vi "Window-Simple Timelapse Player.vi"() -> ()   [LabVIEW 2013]
uses:
  User Interface/Visualisation/Timelapse Viewer/Typedefs/Custom slider-vertical.ctl
  User Interface/Visualisation/Timelapse Viewer/Typedefs/Timelapse viewer refs.ctl
  <vilib>/Utility/miscctls.llb/LVPointTypeDef.ctl
  User Interface/Visualisation/Timelapse Viewer/Typedefs/Speed Viewer States enum.ctl
  Typedefs/Save-Load enum.ctl
  User Interface/Visualisation/Functional Imaging Viewer/Typedefs/Get-Set-Clear Control.ctl
  User Interface/Visualisation/Timelapse Viewer/Typedefs/Select Play-Stop button to show.ctl
  <vilib>/vision/Image Controls.llb/IMAQ Image.ctl
  User Interface/Visualisation/Timelapse Viewer/Globals/gl_Time series viewer globals.vi
  Global Variables/General Globals.vi
panel:
  in  "Intensity":T1={-4095.0, 4095.0} scale=0.0..4095.0
  in  "Back":bool
  in  "Play":bool
  in  "Stop":bool
  in  "Colour":u16(ring)=2 items=["Gray", "Red", "Green"]
  out "Image":T2(plugin-control)
  in  "AVI File Path":path
  out "Speed Graph":dbl[](graph) caption="Speed Chart"
  out "Export data subset":bool
  out "Export vid":bool
  out "Stop (ind)":bool
  in  "Scrollbar":i32(c297)
  out "Speed Profile Graph":dbl[](graph)
  # "<-- Available through the menu"
  # "<-- Available through the menu"
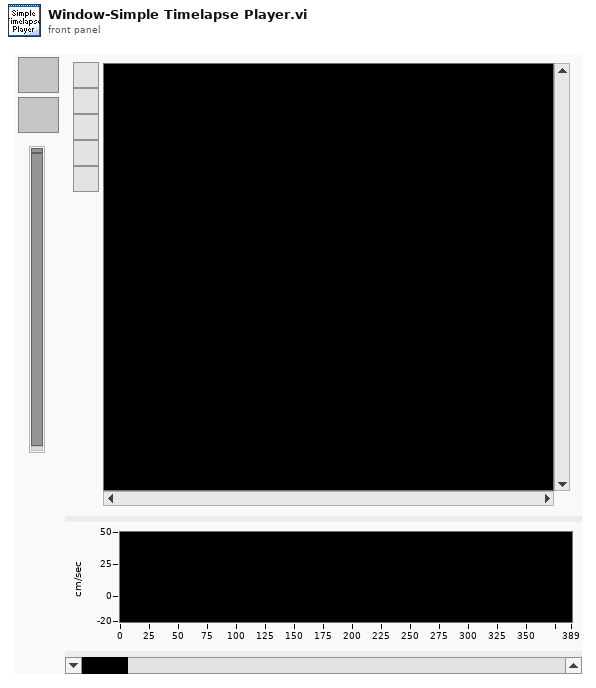
[diagram p1: front panel]
types:
  T1 = typedef "Custom slider-vertical.ctl" = cluster{dbl, dbl}
  T2 = typedef "IMAQ Image.ctl" = refnum<image>
  T3 = typedef "Timelapse viewer refs.ctl" = cluster{"This VI":refnum<vi>, "AVI Mode ind":refnum<vi>, "Play":refnum<vi>, "Stop":refnum<vi>, "Back":refnum<vi>, "Scrollbar":refnum<vi>, "Video length info":refnum<vi>, "Expected speed values":refnum<vi>, "Intensity":refnum<vi>, "Path":refnum<vi>, "Selection sliders":refnum<vi>, "Speed Graph ref":refnum<vi>, "Frame rate set (fps)":refnum<vi>}
  T4 = typedef "LVPointTypeDef.ctl" = cluster{"Horizontal":i16, "Vertical":i16}
  T5 = typedef "Save-Load enum.ctl" = enum16{"Save to file", "Load from file", "Compare from file"}
  T6 = typedef "Speed Viewer States enum.ctl" = enum16{"Idle", "Initialise", "Playback", "Scroll bar event", "Speed cursor event", "Back to start", "Exit"}
  T7 = typedef "Image Type" = u32
  T8 = typedef "Custom slider-horisontal.ctl" = cluster{dbl, dbl}
  T9 = typedef "Select Play-Stop button to show.ctl" = enum16{"Show Play button", "Show Stop button"}
  T10 = cluster{"Conversion Method":u32, "Minimum Value":i32, "Maximum Value":i32, "Number Of Shifts":i32}
  T11 = typedef "AVI modes refs cluster.ctl" = cluster{"AVI1 ref":T12, "AVI2 refs":T13[], "AVI # frames":u32[]}
  T12 = typedef "AviRefnum.ctl" = refnum<k1>
  T13 = typedef "IMAQ AVI2 Refnum.ctl" = refnum<k20>
  T14 = typedef "AVI implementation enum.ctl" = enum16{"AVI1", "AVI2"}
  T15 = cluster{"# of frames to export":i32, "Initial frame's owning file":T13, "8-bit AVI file path":path, "Cursors location":cluster{"Number of first frame":i32, "Number of last frame":i32}}
  T16 = typedef "Get-Set-Clear Control.ctl" = enum16{"Get", "Set", "Clear"}
  T17 = typedef "Speed graph behaviour enum.ctl" = enum16{"Scrolling data", "Scrolling cursor"}
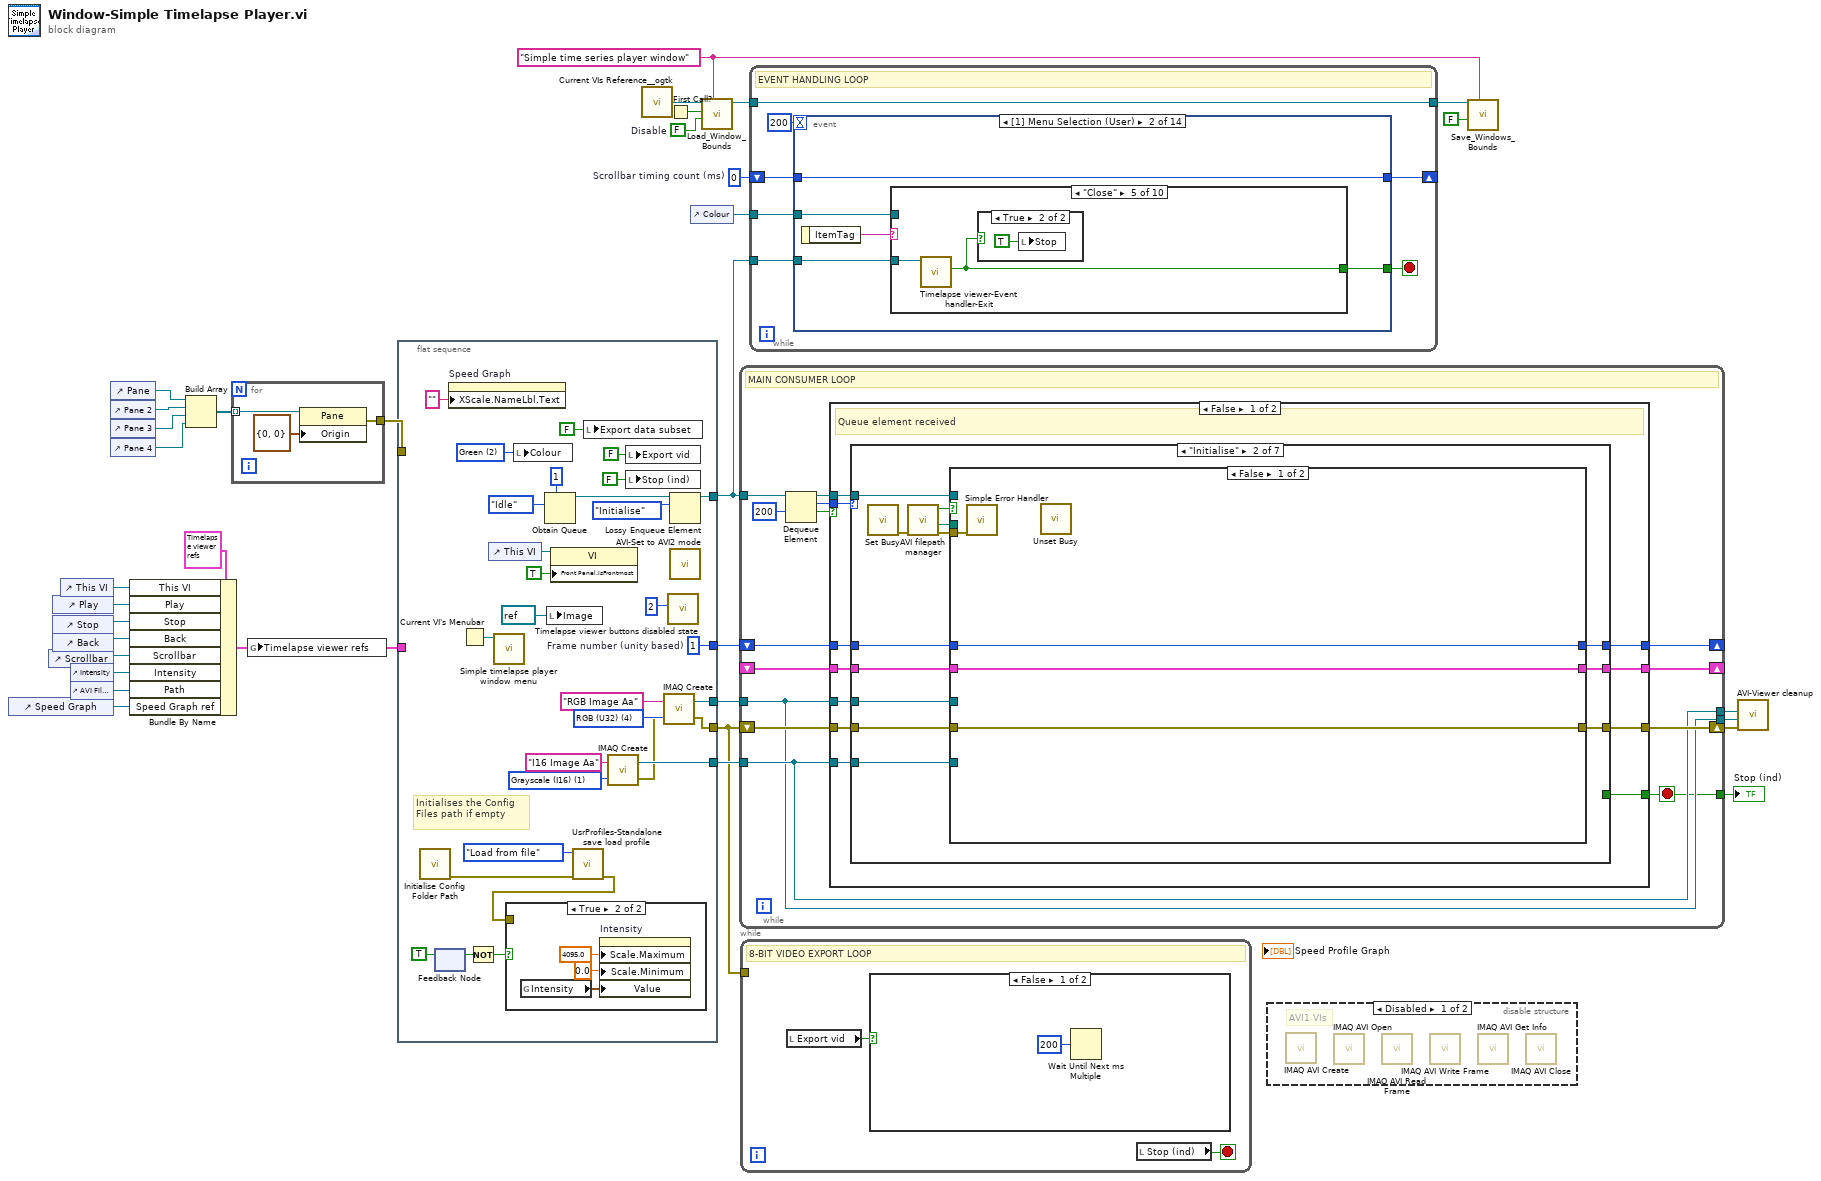
[diagram p0: block diagram]
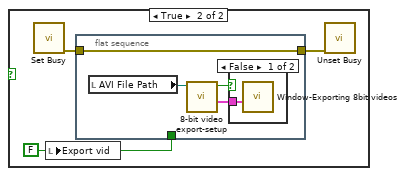
[diagram p3: hidden frame]
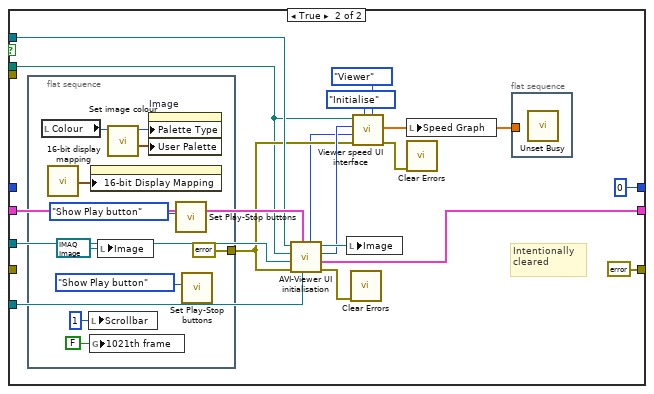
[diagram p7: hidden frame]
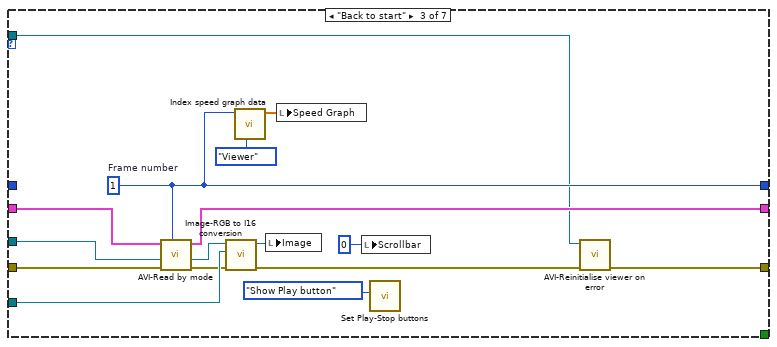
[diagram p8: hidden frame]
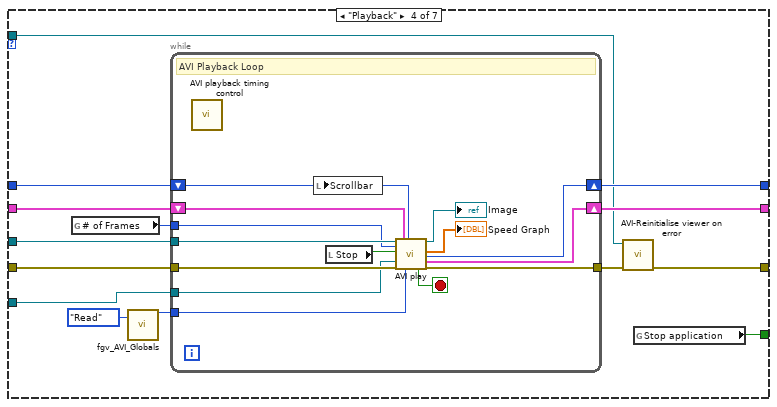
[diagram p9: hidden frame]
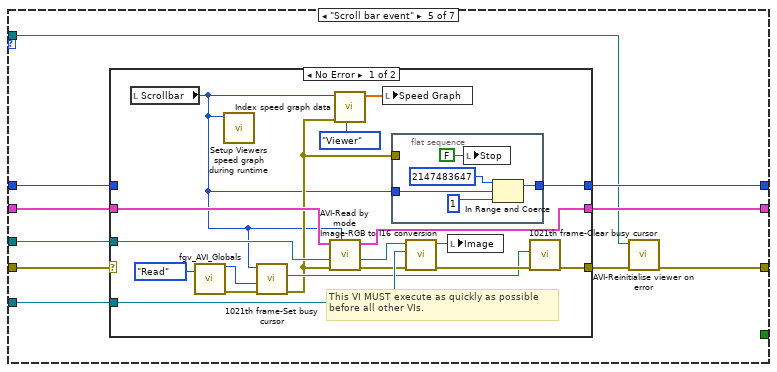
[diagram p10: hidden frame]
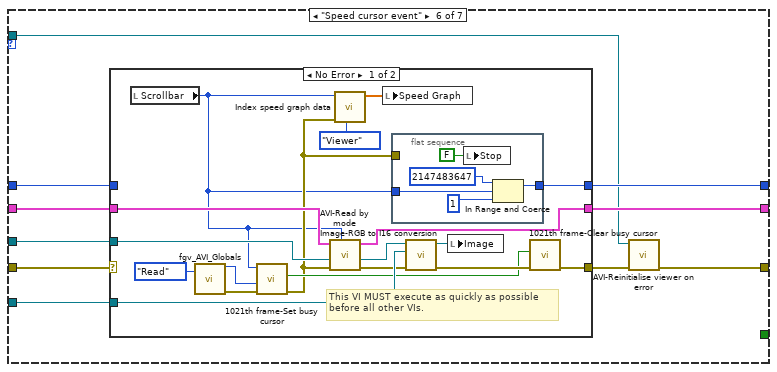
[diagram p12: hidden frame]
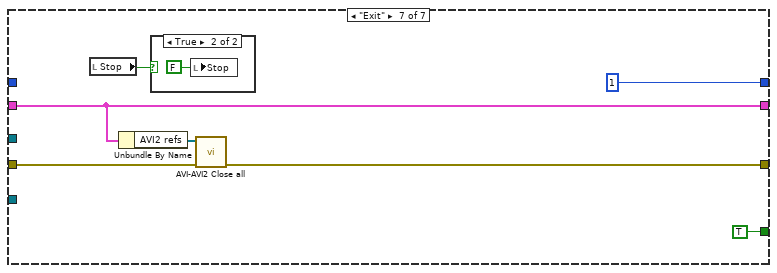
[diagram p14: hidden frame]
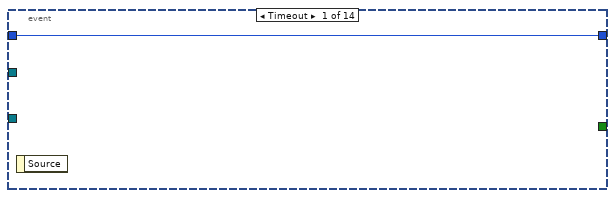
[diagram p17: hidden frame]
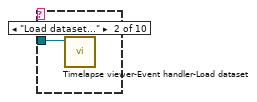
[diagram p19: hidden frame]
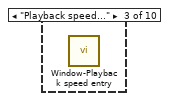
[diagram p20: hidden frame]
diagram:
  w6 = FALSE  # Disable
  w5 = "Simple time series player window" ("Window Name (i.e. Key)")
  w22 = u32 0  # Scrollbar timing count (ms)
  n1 = control-ref of="Speed Graph"() -> (w1:refnum<vi>)
  n2 = control-ref of="Scrollbar"() -> (w24:refnum<vi>)
  n3 = control-ref of="Play"() -> (w27:refnum<vi>)
  n4 = control-ref of="Stop"() -> (w26:refnum<vi>)
  n5 = control-ref of="Back"() -> (w25:refnum<vi>)
  n6 = control-ref of="This VI"() -> (w16:refnum<vi>)
  n7 = control-ref of="Intensity"() -> (w23:refnum<vi>)
  n8 = control-ref of="AVI File Path"() -> (w21:refnum<vi>)
  n9 = control-ref of="Pane"() -> (w14:refnum<vi>)
  n10 = control-ref of="Pane 2"() -> (w13:refnum<vi>)
  n11 = control-ref of="Pane 3"() -> (w12:refnum<vi>)
  n12 = control-ref of="Pane 4"() -> (w11:refnum<vi>)
  n13 = Bundle By Name(cluster=T3 {"This VI"=refnum, "AVI Mode ind"=refnum, "Play"=refnum, "Stop"=refnum, "Back"=refnum, "Scrollbar"=refnum, "Video length info"=refnum, "Expected speed values"=refnum, "Intensity"=refnum, "Path"=refnum, "Selection sliders"=refnum, "Speed Graph ref"=refnum, "Frame rate set (fps)"=refnum}, "This VI"=w16, "Play"=w27, "Stop"=w26, "Back"=w25, "Scrollbar"=w24, "Intensity"=w23, "Path"=w21, "Speed Graph ref"=w1) -> (w19:T3)
  n14 = Build Array(w14, w13, w12, w11) -> (w10:refnum<vi>[])
  n15 = for {
    tunnel: w10 -> [w36] mode=indexing
    tunnel: [w35] -> w9
    n16 = property class="Pane"(reference=w36, "Origin"=T4 {"Horizontal"=0, "Vertical"=0}) -> (error out=w35:errorcluster)  [unwired: 1 in, 1 out]
  }
  n17 = global write "gl_Time series viewer globals.vi" "Timelapse viewer refs"(w19) -> ()
  n18 = flat-sequence {
    tunnel: [w65] -> w34
    tunnel: [w62] -> w33
    tunnel: [w54] -> w17
    tunnel: [w58] -> w31
    tunnel: [w56] -> w30
    tunnel: w19 -> [_]
    tunnel: w9 -> [_]
    frame #0 {
      w47 = u16 2 items=["Gray", "Red", "Green"] ("Colour")
      w56 = 1  # Frame number (unity based)
      w64 = T7 1 items=["Grayscale (U8)", "Grayscale (I16)", "Grayscale (SGL)", "Complex (CSG)", "RGB (U32)", "HSL (U32)", "RGB (U64)", "Grayscale (U16)"] ("Image Type")
      w66 = T7 4 items=["Grayscale (U8)", "Grayscale (I16)", "Grayscale (SGL)", "Complex (CSG)", "RGB (U32)", "HSL (U32)", "RGB (U64)", "Grayscale (U16)"] ("Image Type")
      # "Initialises the Config Files path if empty"
      n19 = call "Initialise Config Folder Path.vi"() -> ("error out"=w43:errorcluster)  [unwired: 9 in, 2 out]
      n20 = feedback #1() -> (w39:bool)  [unwired: 1 in]
      n21 = feedback-in #1(TRUE) -> ()
      n22 = property on="Speed Graph" class="WFGraph (strict)"("XScale.NameLbl.Text"="" ("X Scale.Name Label.Text")) -> ()  [unwired: 2 in, 2 out]
      n23 = Current VI's Menubar() -> (w48:refnum<k9>)
      n24 = Not(x=w39) -> (.not. x?=w42:bool)
      n25 = control-ref of="This VI"() -> (w52:refnum<vi>)
      n26 = call "Simple timelapse player window menu.vi"("menu"=w48) -> ()  [unwired: 9 in, 2 out]
      n27 = local write "Colour"(w47) -> ()
      n28 = Obtain Queue(max queue size (-1, unlimited)=1, element data type=Speed_Viewer_States_enum."Idle" ("States")) -> (queue out=w59:refnum<queue>)  [unwired: 3 in, 2 out]
      n29 = local write "Image"(refnum<image> refnum ("New Image")) -> ()
      n30 = property on="Property Node" class="VI"(reference=w52, "Front Panel.IsFrontmost"=TRUE ("Front Panel Window:Is Frontmost")) -> ()  [unwired: 1 in, 2 out]
      n31 = call "UsrProfiles-Standalone save load profile.vi"("Error in"=w43, "Function"=Save-Load_enum."Load from file") -> ("error out"=w41:errorcluster)  [unwired: 9 in]
      n32 = case shown="True" w42 {
        tunnel: w41 -> [_ _]
        frame False {
        }
        frame True {
          n33 = global read "gl_Time series viewer globals.vi" "Intensity"() -> (w68:T8)
          n34 = property on="Intensity" class="Slide (strict)"("Scale.Maximum"=4095.0 ("Scale.Range:Maximum"), "Scale.Minimum"=0.0 ("Scale.Range:Minimum"), "Value"=w68) -> ()  [unwired: 2 in, 2 out]
        }
      }
      n35 = local write "Export data subset"(FALSE ("Export data subset")) -> ()
      n36 = call "IMAQ Create"("Image Name"="I16 Image Aa", "Image Type"=w64) -> ("New Image"=w62:T2, "error out"=w55:errorcluster)  [unwired: 2 in, 1 out]
      n37 = local write "Export vid"(FALSE ("Export")) -> ()
      n38 = local write "Stop (ind)"(FALSE ("Boolean")) -> ()
      n39 = call "IMAQ Create"("Image Name"="RGB Image Aa", "Image Type"=w66, "error in (no error)"=w55) -> ("New Image"=w65:T2, "error out"=w54:errorcluster)  [unwired: 1 in, 1 out]
      n40 = call "Timelapse viewer buttons disabled state.vi"("Disabled"=2) -> ()  [unwired: 10 in, 1 out]
      n41 = Lossy Enqueue Element(queue=w59, element=Speed_Viewer_States_enum."Initialise" ("States")) -> (queue out=w58:refnum<queue>)  [unwired: 1 in, 3 out]
      n42 = call "AVI-Set to AVI2 mode.vi"() -> ()  [unwired: 11 in, 1 out]
    }
  }
  n43 = call "Current VIs Reference__ogtk.vi"() -> ("Current VI's reference"=w8:refnum<vi>)  [unwired: 5 in]
  n44 = First Call?() -> (First Call?: T/F=w7:bool)
  n45 = control-ref of="Colour"() -> (w15:refnum<vi>)
  n46 = call "Load_Window_Bounds.vi"("Window Name (i.e. Key)"=w5, "Disable"=w6, "First Call"=w7, "Window VI's Ref"=w8) -> ("reference out"=w3:refnum<vi>)  [unwired: 4 in, 3 out]
  n47 = while {
    tunnel: w34 -> [w73]
    tunnel: w33 -> [w74]
    tunnel: [w74] -> w32
    shift-right: [w81] -> _
    shift-left: w30 -> [w80]
    tunnel: w31 -> [w79]
    shift-right: [w75] -> _
    shift-left: _ -> [w84]
    tunnel: [w73] -> w20
    shift-right: [w82] -> w28
    shift-left: w17 -> [w83]
    tunnel: [w71] -> w18
    stop <- w71 stop-if-true
    # "MAIN CONSUMER LOOP"
    n48 = Dequeue Element(queue=w79, timeout in ms (-1)=200) -> (queue out=w72:refnum<queue>, element=w76:T6, timed out?=w77:bool)  [unwired: 1 in, 1 out]
    n49 = case shown="False" w77 {
      tunnel: w84 -> [w95 w268]
      tunnel: [w94 w268] -> w75
      tunnel: w73 -> [w93 _]
      tunnel: w74 -> [w92 _]
      tunnel: w83 -> [w91 w267]
      tunnel: [w90 w267] -> w82
      tunnel: [w89 w269] -> w81
      tunnel: w80 -> [w88 w269]
      tunnel: w76 -> [w87 _]
      tunnel: [w86 _] -> w71
      tunnel: w72 -> [w85 _]
      frame False {
        # "Queue element received"
        n50 = case shown="\"Initialise\"" w87 {
          tunnel: w95 -> [w97 w111 w156 w172 w192 w228 w261]
          tunnel: [w97 w107 w155 w166 w194 w230 w261] -> w94
          tunnel: w93 -> [_ w106 w153 w171 w193 w229 _]
          tunnel: w92 -> [_ w105 w154 w170 w196 w232 _]
          tunnel: w91 -> [w96 w109 w151 w169 w191 w227 w260]
          tunnel: [w96 w108 w146 w165 w189 w225 w259] -> w90
          tunnel: [w98 w110 w148 w168 w195 w231 1 ("Slide")] -> w89
          tunnel: w88 -> [w98 w104 _ w167 w190 w226 _]
          tunnel: [_ _ _ w159 _ _ TRUE] -> w86
          tunnel: w85 -> [_ w100 w145 w163 w187 w223 _]
          frame Default {
          }
          frame "Initialise" {
            n51 = call <vilib>:"Set Busy.vi"() -> ("error out"=w99:errorcluster)  [unwired: 10 in, 1 out]
            n52 = call "AVI filepath manager.vi"("error in (no error)"=w99) -> ("error"=w101:errorcluster, "AVI File Path"=w102:path, "File path OK"=w103:bool)  [unwired: 8 in]
            n53 = case shown="False" w103 {
              tunnel: w111 -> [w114 w132]
              tunnel: [w115 0] -> w110
              tunnel: w102 -> [_ w122]
              tunnel: w109 -> [w113 _]
              tunnel: [w113 errorcluster {"status"=FALSE, "code"=0, "source"=""} ("error out")] -> w108
              tunnel: [w114 w125] -> w107
              tunnel: w106 -> [_ w124]
              tunnel: w105 -> [_ w130]
              tunnel: w104 -> [w115 _]
              tunnel: w101 -> [w112 _]
              tunnel: w100 -> [_ w128]
              frame False {
                n54 = call <vilib>:"Simple Error Handler.vi"("error in (no error)"=w112) -> ()  [unwired: 4 in, 5 out]
                n55 = call <vilib>:"Unset Busy.vi"() -> ()  [unwired: 11 in, 1 out]
              }
              frame True {
                # "Intentionally cleared"
                n56 = flat-sequence {
                  tunnel: [errorcluster {"status"=FALSE, "code"=0, "source"=""} ("error out")] -> w123
                  frame #0 {
                    n57 = local read "Colour"() -> (w137:u16)
                    n58 = call "16-bit display mapping.vi"() -> ("16-bit Display Mapping"=w136:T10)  [unwired: 10 in, 1 out]
                    n59 = local write "Scrollbar"(1 ("Scrollbar")) -> ()
                    n60 = global write "gl_Time series viewer globals.vi" "1021th frame"(FALSE ("1021th frame")) -> ()
                    n61 = property on="Image" class="ImageControl"("16-bit Display Mapping"=w136) -> ()  [unwired: 2 in, 2 out]
                    n62 = local write "Image"(T2 refnum ("New Image")) -> ()
                    n63 = call "Set image colour.vi"("Left Image Palette"=w137) -> ("Color Palette"=w139:cluster{"Red":u8, "Green":u8, "Blue":u8}[], "Palette Type"=w138:u32)  [unwired: 9 in]
                    n64 = property on="Image" class="ImageControl"("Palette Type"=w138, "User Palette"=w139) -> ()  [unwired: 2 in, 2 out]
                    n65 = call "Set Play-Stop buttons.vi"("Function"=Select_Play-Stop_button_to_show."Show Play button") -> ()  [unwired: 10 in, 1 out]
                    n66 = call "Set Play-Stop buttons.vi"("Function"=Select_Play-Stop_button_to_show."Show Play button") -> ()  [unwired: 10 in, 1 out]
                  }
                }
                n67 = call "AVI-Viewer UI initialisation.vi"("I16 image ref in"=w130, "AVI modes refs in"=w132, "error in (no error)"=w123, "RGB image ref in"=w124, "AVI File Path"=w122, "Queue in"=w128) -> ("error out"=w117:errorcluster, "AVI modes refs out"=w125:T11, "Number of Frames"=w126:u32, "Refnum out"=w127:T2, "Scrollbar position"=w119:i32)  [unwired: 1 in]
                n68 = local write "Image"(w127) -> ()
                n69 = call <vilib>:"Clear Errors.vi"("error in (no error)"=w117) -> ()  [unwired: 6 in, 1 out]
                n70 = call "Viewer speed UI interface.vi"("Caller"=enum16{"Viewer", "Exporter"}."Viewer", "Function"=enum16{"Initialise", "Update"}."Initialise", "error in (no error)"=w123, "Gobal frame number in Timelapse data/master video (1 based)"=w119, "Number of Frames"=w126, "Speed Data folder path+dummy filename"=w122) -> ("error out"=w121:errorcluster, "Speed waveform graph data"=w116:dbl[])  [unwired: 2 in, 2 out]
                n71 = local write "Speed Graph"(w116) -> ()
                n72 = call <vilib>:"Clear Errors.vi"("error in (no error)"=w121) -> ()  [unwired: 6 in, 1 out]
                n73 = flat-sequence {
                  tunnel: w116 -> [_]
                  frame #0 {
                    n74 = call <vilib>:"Unset Busy.vi"() -> ()  [unwired: 11 in, 1 out]
                  }
                }
              }
            }
          }
          frame "Back to start" {
            w148 = 1  # Frame number
            n75 = call "AVI-Read by mode.vi"("Frame number (unity-based)"=w148, "error in (no error)"=w151, "RGB image ref in"=w153, "AVI modes refs"=w156) -> ("error out"=w150:errorcluster, "RGB image ref out"=w157:T2, "AVI modes refs"=w155:T11)  [unwired: 5 in]
            n76 = call "Image-RGB to I16 conversion.vi"("error in (no error)"=w150, "I16 image ref in"=w154, "RGB image ref in"=w157) -> ("error out"=w147:errorcluster, "I16 image ref out"=w152:T2)  [unwired: 7 in]
            n77 = call "Index speed graph data.vi"("Caller"=enum16{"Viewer", "Exporter"}."Viewer", "Gobal frame number in Timelapse data/master video (1 based)"=w148) -> ("Speed data waveform graph"=w143:dbl[])  [unwired: 7 in, 2 out]
            n78 = local write "Image"(w152) -> ()
            n79 = local write "Speed Graph"(w143) -> ()
            n80 = local write "Scrollbar"(0 ("Scrollbar")) -> ()
            n81 = call "Set Play-Stop buttons.vi"("Function"=Select_Play-Stop_button_to_show."Show Play button") -> ()  [unwired: 10 in, 1 out]
            n82 = call "AVI-Reinitialise viewer on error.vi"("error in (no error)"=w147, "Queue in"=w145) -> ("error out"=w146:errorcluster)  [unwired: 9 in]
          }
          frame "Playback" {
            n83 = global read "gl_Time series viewer globals.vi" "# of Frames"() -> (w160:u32)
            n84 = call "fgv_AVI_Globals.vi"("Function"=enum16{"Intialize", "Write", "Read", "Clear"}."Read") -> ("AVI mode"=w161:T14)  [unwired: 11 in, 3 out]
            n85 = while {
              tunnel: w171 -> [w184]
              tunnel: w170 -> [w176]
              tunnel: w169 -> [w182]
              tunnel: [w183] -> w164
              shift-right: [w180] -> w168
              shift-left: w167 -> [w181]
              shift-right: [w185] -> w166
              shift-left: w172 -> [w186]
              tunnel: w161 -> [w178]
              tunnel: w160 -> [w175]
              stop <- w179 stop-if-true
              # "AVI Playback Loop"
              n86 = call "AVI playback timing control.vi"() -> ()  [unwired: 8 in, 4 out]
              n87 = local write "Scrollbar"(w181) -> ()
              n88 = local read "Stop"() -> (w177:bool)
              n89 = call "AVI play.vi"("RGB Image ref"=w184, "Number of Frames"=w175, "Stop button pressed"=w177, "I16 Image ref"=w176, "error in (no error)"=w182, "AVI modes refs in"=w186, "AVI mode"=w178, "Frame number (in)"=w181) -> ("Playback stopped"=w179:bool, "I16 image ref out"=→"Image":T2, "Speed data waveform graph"=→"Speed Graph":dbl[], "Frame number (out)"=w180:i32, "AVI modes refs out"=w185:T11, "error out"=w183:errorcluster)  [unwired: 6 in]
            }
            n90 = call "AVI-Reinitialise viewer on error.vi"("error in (no error)"=w164, "Queue in"=w163) -> ("error out"=w165:errorcluster)  [unwired: 9 in]
            n91 = global read "General Globals.vi" "Stop application"() -> (w159:bool)
          }
          frame "Scroll bar event" {
            n92 = case shown="No Error" w191 {
              selector: w191 -> [_ w222]
              tunnel: w196 -> [w214 _]
              tunnel: [w212 w221] -> w195
              tunnel: [w201 w220] -> w194
              tunnel: w193 -> [w210 _]
              tunnel: w192 -> [w208 w220]
              tunnel: [w203 w222] -> w188
              tunnel: w190 -> [_ w221]
              frame No Error {
                # "This VI MUST execute as quickly as possible\nbefore all other VIs."
                n93 = local read "Scrollbar"() -> (w197:i32)
                n94 = call "fgv_AVI_Globals.vi"("Function"=enum16{"Intialize", "Write", "Read", "Clear"}."Read") -> ("AVI mode"=w206:T14, "error out"=w205:errorcluster)  [unwired: 11 in, 2 out]
                n95 = call "Setup Viewers speed graph during runtime.vi"("Frame number"=w197) -> ()  [unwired: 10 in, 1 out]
                n96 = call "1021th frame-Set busy cursor.vi"("error in (no error)"=w205, "AVI mode"=w206, "Frame number"=w197) -> ("error out"=w200:errorcluster, "Busy cursor was set"=w202:bool)  [unwired: 7 in]
                n97 = call "AVI-Read by mode.vi"("Frame number (unity-based)"=w197, "error in (no error)"=w200, "RGB image ref in"=w210, "AVI modes refs"=w208) -> ("error out"=w211:errorcluster, "RGB image ref out"=w209:T2, "AVI modes refs"=w201:T11)  [unwired: 5 in]
                n98 = call "Index speed graph data.vi"("Caller"=enum16{"Viewer", "Exporter"}."Viewer", "error in (no error)"=w200, "Gobal frame number in Timelapse data/master video (1 based)"=w197) -> ("Speed data waveform graph"=w198:dbl[])  [unwired: 6 in, 2 out]
                n99 = local write "Speed Graph"(w198) -> ()
                n100 = flat-sequence {
                  tunnel: [w217] -> w212
                  tunnel: w197 -> [w215]
                  tunnel: w200 -> [_]
                  frame #0 {
                    n101 = local write "Stop"(FALSE ("Stop")) -> ()
                    n102 = In Range and Coerce(upper limit=2147483647, x=w215, lower limit=1) -> (coerced(x)=w217:i32)  [unwired: 1 out]
                  }
                }
                n103 = call "Image-RGB to I16 conversion.vi"("error in (no error)"=w211, "I16 image ref in"=w214, "RGB image ref in"=w209) -> ("error out"=w204:errorcluster, "I16 image ref out"=w213:T2)  [unwired: 7 in]
                n104 = local write "Image"(w213) -> ()
                n105 = call "1021th frame-Clear busy cursor.vi"("error in (no error)"=w204, "Busy cursor was set"=w202) -> ("error out"=w203:errorcluster)  [unwired: 9 in]
              }
              frame Error {
              }
            }
            n106 = call "AVI-Reinitialise viewer on error.vi"("error in (no error)"=w188, "Queue in"=w187) -> ("error out"=w189:errorcluster)  [unwired: 9 in]
          }
          frame "Speed cursor event" {
            n107 = case shown="No Error" w227 {
              selector: w227 -> [_ w258]
              tunnel: w232 -> [w250 _]
              tunnel: [w248 w257] -> w231
              tunnel: [w237 w256] -> w230
              tunnel: w229 -> [w246 _]
              tunnel: w228 -> [w244 w256]
              tunnel: [w239 w258] -> w224
              tunnel: w226 -> [_ w257]
              frame No Error {
                # "This VI MUST execute as quickly as possible\nbefore all other VIs."
                n108 = local read "Scrollbar"() -> (w233:i32)
                n109 = call "fgv_AVI_Globals.vi"("Function"=enum16{"Intialize", "Write", "Read", "Clear"}."Read") -> ("AVI mode"=w242:T14, "error out"=w241:errorcluster)  [unwired: 11 in, 2 out]
                n110 = call "1021th frame-Set busy cursor.vi"("error in (no error)"=w241, "AVI mode"=w242, "Frame number"=w233) -> ("error out"=w236:errorcluster, "Busy cursor was set"=w238:bool)  [unwired: 7 in]
                n111 = call "AVI-Read by mode.vi"("Frame number (unity-based)"=w233, "error in (no error)"=w236, "RGB image ref in"=w246, "AVI modes refs"=w244) -> ("error out"=w247:errorcluster, "RGB image ref out"=w245:T2, "AVI modes refs"=w237:T11)  [unwired: 5 in]
                n112 = call "Index speed graph data.vi"("Caller"=enum16{"Viewer", "Exporter"}."Viewer", "error in (no error)"=w236, "Gobal frame number in Timelapse data/master video (1 based)"=w233) -> ("Speed data waveform graph"=w234:dbl[])  [unwired: 6 in, 2 out]
                n113 = local write "Speed Graph"(w234) -> ()
                n114 = flat-sequence {
                  tunnel: [w253] -> w248
                  tunnel: w233 -> [w251]
                  tunnel: w236 -> [_]
                  frame #0 {
                    n115 = local write "Stop"(FALSE ("Stop")) -> ()
                    n116 = In Range and Coerce(upper limit=2147483647, x=w251, lower limit=1) -> (coerced(x)=w253:i32)  [unwired: 1 out]
                  }
                }
                n117 = call "Image-RGB to I16 conversion.vi"("error in (no error)"=w247, "I16 image ref in"=w250, "RGB image ref in"=w245) -> ("error out"=w240:errorcluster, "I16 image ref out"=w249:T2)  [unwired: 7 in]
                n118 = local write "Image"(w249) -> ()
                n119 = call "1021th frame-Clear busy cursor.vi"("error in (no error)"=w240, "Busy cursor was set"=w238) -> ("error out"=w239:errorcluster)  [unwired: 9 in]
              }
              frame Error {
              }
            }
            n120 = call "AVI-Reinitialise viewer on error.vi"("error in (no error)"=w224, "Queue in"=w223) -> ("error out"=w225:errorcluster)  [unwired: 9 in]
          }
          frame "Exit" {
            n121 = local read "Stop"() -> (w265:bool)
            n122 = Unbundle By Name(w261) -> ("AVI2 refs"=w262:T13[])
            n123 = case shown="True" w265 {
              frame False {
              }
              frame True {
                n124 = local write "Stop"(FALSE ("Stop")) -> ()
              }
            }
            n125 = call "AVI-AVI2 Close all.vi"("error in (no error)"=w260, "AVI2 ref"=w262) -> ("error out"=w259:errorcluster)  [unwired: 9 in]
          }
        }
      }
      frame True {
        # "Timeout"
      }
    }
  }
  "Stop (ind)" <- w18
  n126 = while {
    tunnel: w17 -> [_]
    stop <- w271 stop-if-true
    # "8-BIT VIDEO EXPORT LOOP"
    n127 = local read "Export vid"() -> (w270:bool)
    n128 = case shown="False" w270 {
      frame False {
        n129 = Wait Until Next ms Multiple(millisecond multiple=u32 200) -> ()  [unwired: 1 out]
      }
      frame True {
        w275 = FALSE ("Export")
        n130 = call <vilib>:"Set Busy.vi"() -> ("error out"=w274:errorcluster)  [unwired: 10 in, 1 out]
        n131 = local write "Export vid"(w275) -> ()
        n132 = flat-sequence {
          tunnel: w275 -> [_]
          tunnel: w274 -> [w279]
          tunnel: [w279] -> w273
          frame #0 {
            n133 = local read "AVI File Path"() -> (w278:path)
            n134 = call "8-bit video export-setup.vi"("selected AVI file path"=w278) -> ("output cluster"=w276:T15, "cancelled"=w277:bool)  [unwired: 9 in]
            n135 = case shown="False" w277 {
              tunnel: w276 -> [w280 _]
              frame False {
                n136 = call "Window-Exporting 8bit videos.vi"("Input cluster"=w280) -> ()  [unwired: 11 in]
              }
              frame True {
              }
            }
          }
        }
        n137 = call <vilib>:"Unset Busy.vi"("error in (no error)"=w273) -> ()  [unwired: 10 in, 1 out]
      }
    }
    n138 = local read "Stop (ind)"() -> (w271:bool)
  }
  n139 = while {
    shift-right: [w285] -> _
    shift-left: w22 -> [w284]
    tunnel: w31 -> [w283]
    tunnel: w15 -> [w282]
    tunnel: [w281] -> w2
    tunnel: w3 -> [w281]
    stop <- w286 stop-if-true
    # "EVENT HANDLING LOOP"
    n140 = event shown="[1] Menu Selection (User)" {
      selector: _ -> [_ _ _ _ _ _ _ _ _ _ _ _ _ _]
      dyn-events: _ -> [_ _ _ _ _ _ _ _ _ _ _ _ _ _]
      timeout: 200 -> [_ _ _ _ _ _ _ _ _ _ _ _ _ _]
      tunnel: [_ w290 _ _ _ _ _ _ _ _ _ _ _ w360] -> w286
      tunnel: [w288 w293 w308 w309 w317 w325 w329 w335 w338 w344 w346 w350 w358 w362] -> w285
      tunnel: w284 -> [w288 w293 w308 w311 w317 w325 w329 w335 w338 w344 w346 w350 w358 w362]
      tunnel: w283 -> [_ w291 _ w310 _ w323 _ _ w337 w341 _ w349 _ w361]
      tunnel: w282 -> [_ w289 _ _ _ _ _ _ _ _ _ _ _ _]
      event Timeout {
        n141 = event-data() -> ()  [unwired: 1 in, 1 out]
      }
      event Menu Selection (User) {
        n142 = event-data() -> ("ItemTag"=w292:string)  [unwired: 1 in]
        n143 = case shown="\"Close\"" w292 {
          tunnel: w291 -> [_ w294 _ _ w297 _ _ _ _ _]
          tunnel: [_ _ _ _ w296 _ _ _ _ _] -> w290
          tunnel: w289 -> [_ _ _ _ _ _ _ w302 w304 w306]
          frame Default {
          }
          frame "Load dataset..." {
            n144 = call "Timelapse viewer-Event handler-Load dataset.vi"("queue"=w294) -> ()  [unwired: 11 in]
          }
          frame "Playback speed..." {
            n145 = call "Window-Playback speed entry.vi"() -> ()  [unwired: 10 in, 2 out]
          }
          frame "Original speed (x1)" {
            n146 = flat-sequence {
              frame #0 {
                n147 = global write "gl_Time series viewer globals.vi" "Use manual FPS?"(FALSE ("Use manual FPS?")) -> ()
              }
              frame #1 {
                n148 = call "AVI playback timing control.vi"() -> ()  [unwired: 8 in, 4 out]
              }
            }
          }
          frame "Close" {
            n149 = call "Timelapse viewer-Event handler-Exit.vi"("Queue in"=w297) -> ("Exit"=w296:bool)  [unwired: 10 in]
            n150 = case shown="True" w296 {
              frame False {
              }
              frame True {
                n151 = local write "Stop"(TRUE ("Stop")) -> ()
              }
            }
          }
          frame "Export 8-bit video file..." {
            "Export vid" <- TRUE
          }
          frame "Export time-lapse subset..." {
            "Export data subset" <- TRUE
          }
          frame "Red" {
            w301 = u16 1 items=["Gray", "Red", "Green"] ("Colour")
            n152 = property class="Ring (strict)"(reference=w302, "Val(Sgnl)"=w301) -> ()  [unwired: 1 in, 2 out]
          }
          frame "Green" {
            w303 = u16 2 items=["Gray", "Red", "Green"] ("Colour")
            n153 = property class="Ring (strict)"(reference=w304, "Val(Sgnl)"=w303) -> ()  [unwired: 1 in, 2 out]
          }
          frame "Gray" {
            w305 = u16 0 items=["Gray", "Red", "Green"] ("Colour")
            n154 = property class="Ring (strict)"(reference=w306, "Val(Sgnl)"=w305) -> ()  [unwired: 1 in, 2 out]
          }
        }
      }
      event "Scrollbar", "Speed Graph": Shortcut Menu Selection (User) {
        n155 = event-data() -> ("ItemTag"=w307:string)  [unwired: 1 in]
        n156 = call "Timelapse viewer-Shortcut menu handler.vi"("ItemTag"=w307) -> ()  [unwired: 11 in]
      }
      event "Scrollbar": Value Change {
        n157 = event-data() -> ()  [unwired: 1 in, 1 out]
        n158 = call "Event case-Scrollbar value change.vi"("Tick count in"=w311, "Queue in"=w310) -> ("Tick count"=w309:u32)  [unwired: 8 in, 1 out]
      }
      event "Speed Graph": Shortcut Menu Activation? {
        n159 = event-data() -> ("MenuRef"=w312:refnum<k9>)  [unwired: 1 in]
        n160 = call "FGV_Speed graph behaviour-Main viewer.vi"("Function"=Get-Set-Clear_Control."Get") -> ("Speed graph behaviour"=w314:T17)  [unwired: 9 in, 1 out]
        n161 = case shown="\"Scrolling data\", Default" w314 {
          tunnel: [bool[] [FALSE, TRUE] bool[] [TRUE, FALSE]] -> w313
          frame "Scrolling data", Default {
          }
          frame "Scrolling cursor" {
          }
        }
        n162 = for {
          tunnel: string[] ["scrolling cursor", "scrolling data"] -> [w322] mode=indexing
          tunnel: w312 -> [w321]
          tunnel: w313 -> [w320] mode=indexing
          n163 = Set Menu Item Info(6:w320, 7:w322, 11:w321) -> ()  [unwired: 4 in, 2 out]
        }
        n164 = event-data() -> ()  [unwired: 2 in, 1 out]
      }
      event "Speed Graph": Cursor Move; "Speed Graph": Cursor Release {
        n165 = event-data() -> ("CursRef"=w324:refnum<vi>)  [unwired: 1 in]
        n166 = call "Event case-Speed graph cursor moved.vi"("queue in"=w323, "Cursor in"=w324) -> ()  [unwired: 9 in, 1 out]
      }
      event "Speed Graph": event type 3.0.x80000027 {
        n167 = event-data() -> ()  [unwired: 1 in, 1 out]
        n168 = call "FGV_Speed graph behaviour-Main viewer.vi"("Function"=Get-Set-Clear_Control."Get") -> ("Speed graph behaviour"=w328:T17)  [unwired: 9 in, 1 out]
        n169 = case shown="\"Scrolling data\", Default" w328 {
          tunnel: [TRUE FALSE] -> w326
          frame "Scrolling data", Default {
            # "Moving the speed data graph's cursor manually is \nprevented when the mode is \"Scrolling data\"."
          }
          frame "Scrolling cursor" {
            # "Moving the speed data graph's cursor manually is \nallowed when the mode is \"Scrolling cursor\"."
          }
        }
        n170 = event-data("Discard?"=w326) -> ()  [unwired: 1 in, 1 out]
      }
      event "Colour": Value Change {
        n171 = event-data() -> ()  [unwired: 1 in, 1 out]
        n172 = call "Set image colour.vi"("Left Image Palette"="Colour") -> ("Color Palette"=w332:cluster{"Red":u8, "Green":u8, "Blue":u8}[], "Palette Type"=w333:u32)  [unwired: 9 in]
        n173 = property on="Image" class="ImageControl"("Palette Type"=w333, "User Palette"=w332) -> ()  [unwired: 2 in, 2 out]
      }
      event "AVI File Path": Value Change {
        w336 = TRUE ("Stop")
        n174 = event-data() -> ()  [unwired: 1 in, 1 out]
        n175 = local write "Stop"(w336) -> ()
        n176 = flat-sequence {
          tunnel: w337 -> [w340]
          tunnel: w336 -> [_]
          frame #0 {
            n177 = Enqueue Element At Opposite End(queue=w340, element=Speed_Viewer_States_enum."Initialise") -> ()  [unwired: 2 in, 3 out]
          }
        }
      }
      event "Back": Value Change {
        n178 = event-data() -> ()  [unwired: 1 in, 1 out]
        n179 = Enqueue Element At Opposite End(queue=w341, element=Speed_Viewer_States_enum."Back to start") -> ()  [unwired: 2 in, 3 out]
        n180 = local write "Stop"(TRUE ("Stop")) -> ()
      }
      event Value Change {
        n181 = event-data() -> ()  [unwired: 1 in, 1 out]
        n182 = call "16-bit display mapping.vi"() -> ("16-bit Display Mapping"=w345:T10)  [unwired: 10 in, 1 out]
        n183 = property on="Image" class="ImageControl"("16-bit Display Mapping"=w345) -> ()  [unwired: 2 in, 2 out]
      }
      event "Play": Value Change {
        n184 = event-data() -> ()  [unwired: 1 in, 1 out]
        n185 = flat-sequence {
          tunnel: w349 -> [w354]
          tunnel: [w354] -> w348
          tunnel: w348 -> [w355]
          tunnel: [w355] -> w347
          tunnel: w347 -> [w356]
          frame #0 {
            n186 = property on="Speed Graph" class="WFGraph (strict)"("Value"=dbl[] [] ("History Data")) -> ()  [unwired: 2 in, 2 out]
            n187 = local write "Stop"(FALSE ("Stop")) -> ()
            n188 = call "Set Play-Stop buttons.vi"("Function"=Select_Play-Stop_button_to_show."Show Stop button") -> ()  [unwired: 10 in, 1 out]
          }
          frame #1 {
            n189 = call "Set scrollbar at start.vi"("Queue in"=w355) -> ()  [unwired: 10 in, 1 out]
          }
          frame #2 {
            n190 = Enqueue Element(queue=w356, element=Speed_Viewer_States_enum."Playback" ("States")) -> ()  [unwired: 2 in, 3 out]
          }
        }
      }
      event "Stop": Value Change {
        n191 = event-data() -> ()  [unwired: 1 in, 1 out]
      }
      event Panel Close? {
        n192 = event-data() -> ()  [unwired: 1 in, 1 out]
        n193 = call "Timelapse viewer-Event handler-Exit.vi"("Queue in"=w361) -> ("Exit"=w360:bool)  [unwired: 10 in]
        n194 = case shown="True" w360 {
          frame False {
          }
          frame True {
            n195 = local write "Stop"(TRUE ("Stop")) -> ()
          }
        }
        n196 = event-data("Discard?"=TRUE) -> ()  [unwired: 1 in, 1 out]
      }
    }
  }
  n197 = disable-structure shown="Disabled" {
    frame Disabled {
      # "AVI1 VIs"
      n198 = call "IMAQ AVI Create"() -> ()  [unwired: 10 in, 2 out]
      n199 = call "IMAQ AVI Open"() -> ()  [unwired: 10 in, 2 out]
      n200 = call "IMAQ AVI Read Frame"() -> ()  [unwired: 8 in, 4 out]
      n201 = call "IMAQ AVI Write Frame"() -> ()  [unwired: 10 in, 2 out]
      n202 = call "IMAQ AVI Get Info"() -> ()  [unwired: 7 in, 5 out]
      n203 = call "IMAQ AVI Close"() -> ()  [unwired: 11 in, 1 out]
    }
    frame Enabled {
    }
  }
  n204 = call "Save_Windows_Bounds.vi"("Window Name (i.e. Key)"=w5, "Front Panel Window:Open"=FALSE, "Window VI's Ref"=w2) -> ()  [unwired: 8 in, 1 out]
  n205 = call "AVI-Viewer cleanup.vi"("error in (no error)"=w28, "RGB image ref"=w20, "I16 image ref"=w32) -> ()  [unwired: 8 in, 1 out]
